vi "hmi_load_project.vi"(5 "lv-builder.lvlib:lv-builder.lvclass":refnum<class "lv-builder.lvclass">, 7 "hmi_references":T1, 8 "error in (no error)":errorcluster, 11 "build_spec []":T2[](array[typedef])) -> (0 "error out":errorcluster)   [LabVIEW 2015, in "lv-build-interface.lvlib"]
uses:
  lv-build-interface.lvlib
  lv-build/public/_controls/build_specification.ctl
  lv-build/public/_controls/build_type.ctl
  _controls/hmi_references.ctl
  lv-builder/lv-builder.lvclass
  lv-builder/public/accessors/project_file_read.vi
  lv-builder/public/accessors/commit_hash_read.vi
  lv-build/lv-build.lvlib
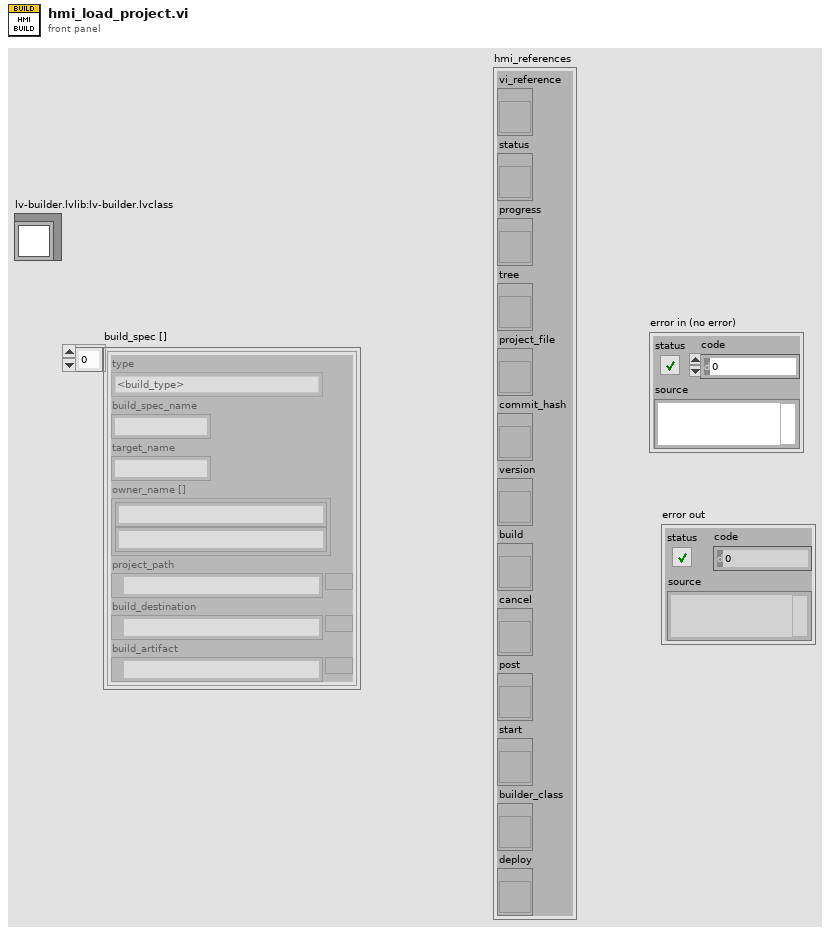
[diagram p1: front panel]
types:
  T1 = typedef "lv-build-interface.lvlib/hmi_references.ctl" = cluster{"vi_reference":refnum<vi>, "status":refnum<vi>, "progress":refnum<vi>, "tree":refnum<vi>, "project_file":refnum<vi>, "commit_hash":refnum<vi>, "version":refnum<vi>, "build":refnum<vi>, "cancel":refnum<vi>, "post":refnum<vi>, "start":refnum<vi>, "builder_class":refnum<vi>, "deploy":refnum<vi>}
  T2 = typedef "lv-build.lvlib/build_specification.ctl" = cluster{"type":T3, "build_spec_name":string, "target_name":string, "owner_name []":string[], "project_path":path, "build_destination":path, "build_artifact":path}
  T3 = typedef "lv-build.lvlib/build_type.ctl" = enum16{"<build_type>", "application_pc", "application_rt", "installer", "llb", "lvlibp", "zip", "fpga", "<null>"}
  T4 = cluster{cluster{"build_spec_name":string, i32}[]}
  T5 = cluster{"target_name":string, "build_spec_name":string, i32}
  T6 = cluster{"target_name":string, "build_spec_name":string, i32}[]
  T7 = cluster{cluster{"build_spec_name":string, i32}[]}[]
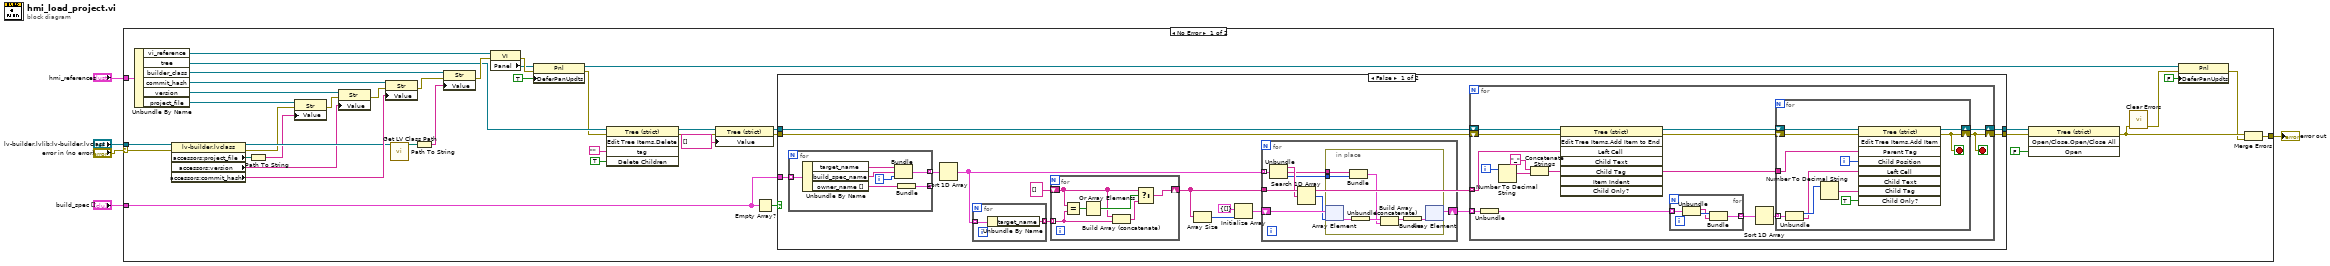
[diagram p0: block diagram]
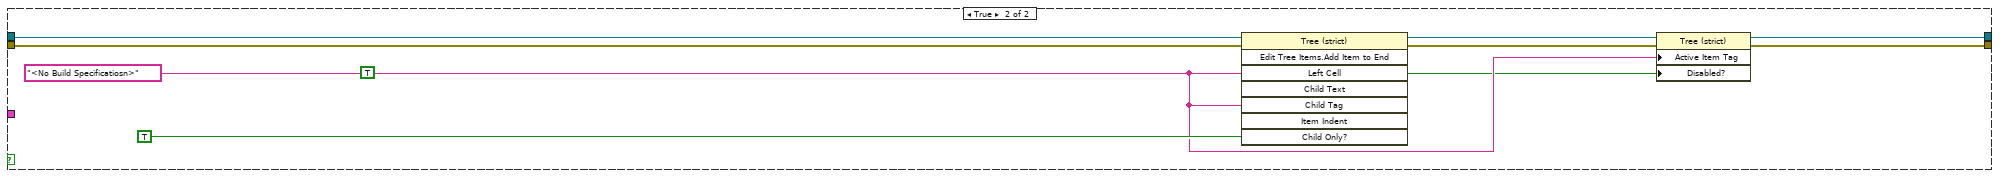
[diagram p2: hidden frame]
diagram:
  n1 = case shown="No Error" "error in (no error)" {
    selector: "error in (no error)" -> [w13 w132]
    tunnel: "hmi_references" -> [w47 _]
    tunnel: "build_spec []" -> [w30 _]
    tunnel: [w23 w132] -> w2
    tunnel: "lv-builder.lvlib:lv-builder.lvclass" -> [w19 _]
    frame No Error {
      n2 = Unbundle By Name(w47) -> ("vi_reference"=w27:refnum<vi>, "tree"=w29:refnum<vi>, "builder_class"=w20:refnum<vi>, "commit_hash"=w18:refnum<vi>, "version"=w21:refnum<vi>, "project_file"=w28:refnum<vi>)
      n3 = property class="lv-builder.lvclass"(reference=w19, error in=w13) -> (reference out=w15:refnum<class "lv-builder.lvclass">, error out=w12:errorcluster, "accessors:project_file"=w6:path, "accessors:version"=w7:string, "accessors:commit_hash"=w17:string)
      n4 = Path To String(path=w6) -> (string=w10:string)
      n5 = property class="Str"(reference=w28, error in=w12, "Value"=w10) -> (error out=w11:errorcluster)  [unwired: 1 out]
      n6 = property class="Str"(reference=w21, error in=w11, "Value"=w7) -> (error out=w16:errorcluster)  [unwired: 1 out]
      n7 = property class="Str"(reference=w18, error in=w16, "Value"=w17) -> (error out=w8:errorcluster)  [unwired: 1 out]
      n8 = call <vilib>:"Get LV Class Path.vi"("object"=w15) -> ("class path"=w14:path)  [unwired: 9 in, 1 out]
      n9 = Path To String(path=w14) -> (string=w9:string)
      n10 = property class="Str"(reference=w20, error in=w8, "Value"=w9) -> (error out=w48:errorcluster)  [unwired: 1 out]
      n11 = property class="VI"(reference=w27, error in=w48) -> (error out=w46:errorcluster, "Panel"=w45:refnum<vi>)  [unwired: 1 out]
      n12 = property class="Pnl"(reference=w45, error in=w46, "DeferPanUpdts"=TRUE ("Defer Panel Updates")) -> (reference out=w42:refnum<vi>, error out=w26:errorcluster)
      n13 = invoke class="Tree (strict)" method="Edit Tree Items.Delete"(reference=w29, error in=w26, "tag"="", "Delete Children"=TRUE ("Delete Children?")) -> (reference out=w34:refnum<vi>, error out=w33:errorcluster)  [unwired: 1 in, 3 out]
      n14 = property class="Tree (strict)"(reference=w34, error in=w33, "Value"=string[] []) -> (reference out=w36:refnum<vi>, error out=w35:errorcluster)
      n15 = Empty Array?(array=w30) -> (empty?=w32:bool)
      n16 = case shown="False" w32 {
        tunnel: [w62 w127] -> w38
        tunnel: [w61 w126] -> w37
        tunnel: w36 -> [w60 w130]
        tunnel: w35 -> [w59 w129]
        tunnel: w30 -> [w58 _]
        frame False {
          n17 = for {
            tunnel: [w75] -> w57 mode=indexing
            tunnel: w58 -> [w74] mode=indexing
            tunnel: [w71] -> _ mode=indexing
            i -> [w73]
            n18 = Unbundle By Name(w74) -> ("target_name"=w77:string, "build_spec_name"=w76:string, "owner_name []"=w72:string[])
            n19 = Bundle("target_name"=w77, "build_spec_name"=w76, w73) -> (w75:T5)  [unwired: 1 in]
            n20 = Bundle("owner_name []"=w72) -> (w71:cluster{"owner_name []":string[]})  [unwired: 1 in]
          }
          n21 = Sort 1D Array(array=w57) -> (sorted array=w53:T6)
          n22 = for {
            tunnel: w53 -> [w70] mode=indexing
            tunnel: [w69] -> w50 mode=indexing
            n23 = Unbundle By Name(w70) -> ("target_name"=w69:string)
          }
          n24 = for {
            shift-right: [w63] -> w49
            shift-left: string[] [] -> [w65]
            tunnel: w50 -> [w67] mode=indexing
            n25 = Equal?(x=w65, y=w67) -> (x = y?=w68:bool[])
            n26 = Or Array Elements(Boolean array=w68) -> (logical OR=w66:bool)
            n27 = Build Array (concatenate)(w65, w67) -> (w64:string[])
            n28 = Select(t=w65, s=w66, f=w64) -> (s? t:f=w63:string[])
          }
          n29 = Array Size(array=w49) -> (size(s)=w55:i32)
          n30 = Initialize Array(T4 {[]}, w55) -> (w54:T7)
          n31 = for {
            shift-right: [w81] -> w52
            shift-left: w54 -> [w83]
            tunnel: w53 -> [w85] mode=indexing
            tunnel: w49 -> [w84]
            n32 = Unbundle(w85) -> ("target_name"=w80:string, "build_spec_name"=w79:string, w78:i32)
            n33 = Search 1D Array(1D array=w84, element=w80) -> (index of element=w82:i32)  [unwired: 1 in]
            n34 = in-place {
              in-place-border: w79 -> [w88]
              in-place-border: w78 -> [w87]
              n35 = in-place-array #1(w83, w82) -> (w92:T4)
              n36 = Bundle("build_spec_name"=w88, w87) -> (w86:cluster{"build_spec_name":string, i32})  [unwired: 1 in]
              n37 = Unbundle(w92) -> (w91:cluster{"build_spec_name":string, i32}[])
              n38 = Build Array (concatenate)(w91, w86) -> (w89:cluster{"build_spec_name":string, i32}[])
              n39 = Bundle(w89) -> (w90:T4)  [unwired: 1 in]
              n40 = in-place-array #1(w90) -> (w81:T7)  [unwired: 1 out]
            }
          }
          n41 = for {
            shift-right: [w103] -> w62
            shift-left: w60 -> [w107]
            shift-right: [w99] -> w61
            shift-left: w59 -> [w106]
            tunnel: w49 -> [w101] mode=indexing
            tunnel: w52 -> [w100] mode=indexing
            i -> [w102]
            stop <- w99 stop-if-true
            n42 = Unbundle(w100) -> (w95:cluster{"build_spec_name":string, i32}[])
            n43 = Number To Decimal String(number=w102) -> (decimal integer string=w97:string)  [unwired: 1 in]
            n44 = Concatenate Strings("_" ("string"), w97) -> (w96:string)
            n45 = invoke class="Tree (strict)" method="Edit Tree Items.Add Item to End"(reference=w107, error in=w106, "Left Cell"=w101, "Child Tag"=w96) -> (reference out=w105:refnum<vi>, error out=w104:errorcluster)  [unwired: 4 in, 6 out]
            n46 = for {
              tunnel: w95 -> [w111] mode=indexing
              tunnel: [w108] -> w94 mode=indexing
              n47 = Unbundle(w111) -> ("build_spec_name"=w109:string, w110:i32)
              n48 = Bundle(w110, "build_spec_name"=w109) -> (w108:cluster{i32, "build_spec_name":string})  [unwired: 1 in]
            }
            n49 = Sort 1D Array(array=w94) -> (sorted array=w93:cluster{i32, "build_spec_name":string}[])
            n50 = for {
              tunnel: w96 -> [w118]
              shift-right: [w120] -> w103
              shift-left: w105 -> [w122]
              shift-right: [w116] -> w99
              shift-left: w104 -> [w121]
              tunnel: w93 -> [w117] mode=indexing
              i -> [w115]
              stop <- w116 stop-if-true
              n51 = Unbundle(w117) -> (w113:i32, "build_spec_name"=w112:string)
              n52 = Number To Decimal String(number=w113) -> (decimal integer string=w114:string)  [unwired: 1 in]
              n53 = invoke class="Tree (strict)" method="Edit Tree Items.Add Item"(reference=w122, error in=w121, "Parent Tag"=w118, "Child Position"=w115, "Left Cell"=w112, "Child Tag"=w114, "Child Only?"=TRUE) -> (reference out=w120:refnum<vi>, error out=w116:errorcluster)  [unwired: 2 in, 7 out]
            }
          }
        }
        frame True {
          w124 = "<No Build Specificatiosn>"
          n54 = invoke class="Tree (strict)" method="Edit Tree Items.Add Item to End"(reference=w130, error in=w129, "Left Cell"=w124, "Child Tag"=w124, "Child Only?"=TRUE) -> (reference out=w128:refnum<vi>, error out=w125:errorcluster)  [unwired: 3 in, 6 out]
          n55 = property class="Tree (strict)"(reference=w128, error in=w125, "Active Item Tag"=w124, "Disabled?"=TRUE ("Active Item:Disabled?")) -> (reference out=w127:refnum<vi>, error out=w126:errorcluster)
        }
      }
      n56 = invoke class="Tree (strict)" method="Open/Close.Open/Close All"(reference=w38, error in=w37, "Open"=FALSE ("Open?")) -> (error out=w25:errorcluster)  [unwired: 1 in, 3 out]
      n57 = call <vilib>:"Clear Errors.vi"("error in (no error)"=w25) -> ("error out"=w22:errorcluster)  [unwired: 5 in, 1 out]
      n58 = property class="Pnl"(reference=w42, error in=w22, "DeferPanUpdts"=FALSE ("Defer Panel Updates")) -> (error out=w24:errorcluster)  [unwired: 1 out]
      n59 = Merge Errors(w25, w24) -> (w23:errorcluster)
    }
    frame Error {
    }
  }
  "error out" <- w2
